vi "Fit.vi"(8 "error in (no error)":errorcluster caption="entrée d'erreur (pas d'erreur)", 10 "y":string[][](array[string]), 11 "LabelBinarizer.lvclass":refnum<class "LabelBinarizer.lvclass">) -> (0 "error out":errorcluster caption="sortie d'erreur", 2 "String Data":string, 3 "LabelBinarizer.lvclass":refnum<class "LabelBinarizer.lvclass">)   [LabVIEW 2020, in "LabelBinarizer.lvclass"]
doc: "Fit label binarizer\n\nReturns : \n\n- String : OK"
uses:
  LabelBinarizer.lvclass
  LabelBinarizer.lvclass/LabelBinarizer.ctl
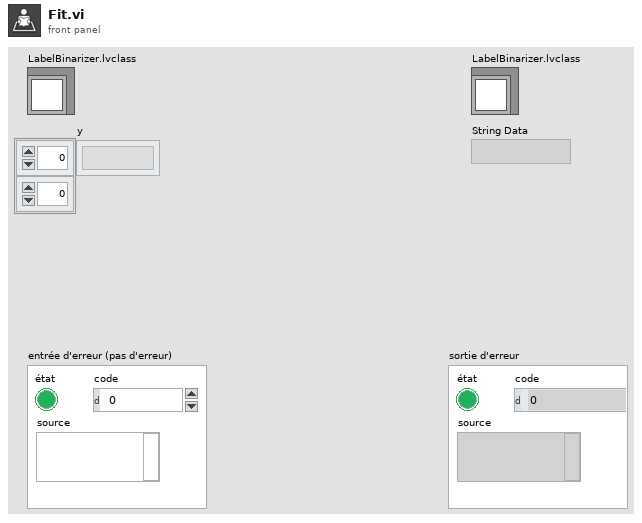
[diagram p1: front panel]
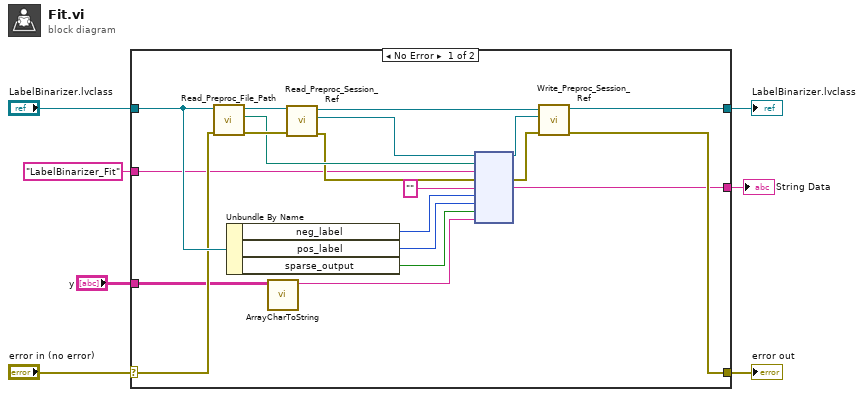
[diagram p0: block diagram]
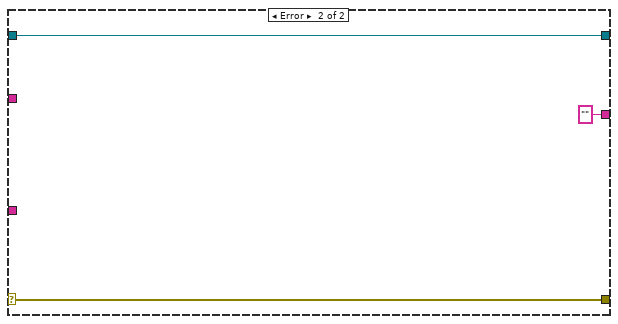
[diagram p2: hidden frame]
diagram:
  n1 = case shown="No Error" "error in (no error)" {
    selector: "error in (no error)" -> [w12 w30]
    tunnel: [w13 w30] -> w6
    tunnel: [w14 w29] -> w4
    tunnel: "LabelBinarizer.lvclass" -> [w15 w29]
    tunnel: "LabelBinarizer_Fit" ("Fonction") -> [w11 _]
    tunnel: [w10 ""] -> w2
    tunnel: "y" -> [w9 _]
    frame No Error {
      n2 = call-dynamic "Read_Preproc_File_Path.vi"("error in (no error)"=w12, "Python in"=w15) -> ("error out"=w26:errorcluster, "File_Path"=w23:path, "Python out"=w27:refnum<class "LabelBinarizer.lvclass">)  [unwired: 7 in]
      n3 = Unbundle By Name(w15) -> ("neg_label"=w18:i32, "pos_label"=w17:i32, "sparse_output"=w16:bool)
      n4 = call "ArrayCharToString.vi"("TAB"=w9) -> ("Instruction"=w8:string)  [unwired: 10 in]
      n5 = call-dynamic "Read_Preproc_Session_Ref.vi"("error in (no error)"=w26, "Python in"=w27) -> ("error out"=w22:errorcluster, "Session_ref"=w24:refnum<k35>, "Python out"=w25:refnum<class "LabelBinarizer.lvclass">)  [unwired: 7 in]
      n6 = node(w24, w23, w11, w22, "", w18, w17, w16, w8) -> (w20:refnum<k35>, w21:errorcluster, w10:string)  [unwired: 4 in, 2 out]
      n7 = call-dynamic "Write_Preproc_Session_Ref.vi"("error in (no error)"=w21, "Session_ref"=w20, "Python in"=w25) -> ("error out"=w13:errorcluster, "Python out"=w14:refnum<class "LabelBinarizer.lvclass">)  [unwired: 7 in]
    }
    frame Error {
    }
  }
  "error out" <- w6
  "LabelBinarizer.lvclass" <- w4
  "String Data" <- w2
